vi "471 flame &mq6 (1).vi"() -> ()   [LabVIEW 2017]
panel:
  out "flame indication":bool
  out "Numeric":dbl
  out "dynamic data type":dbl
  out "flame voltage":dbl
  out "mq6 voltage":dbl
  out "Waveform Chart":dynamicdata(graph)
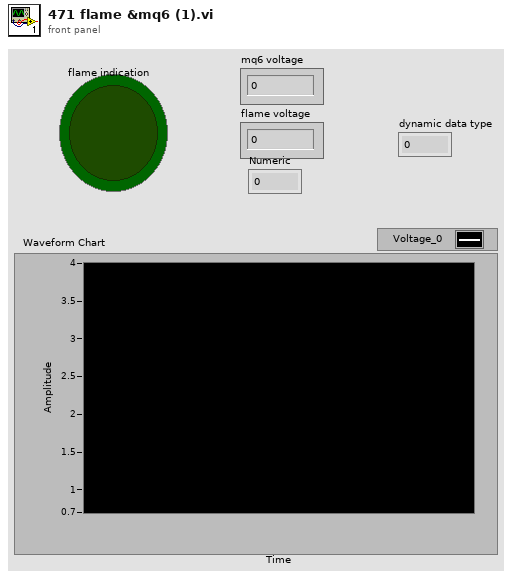
[diagram p1: front panel]
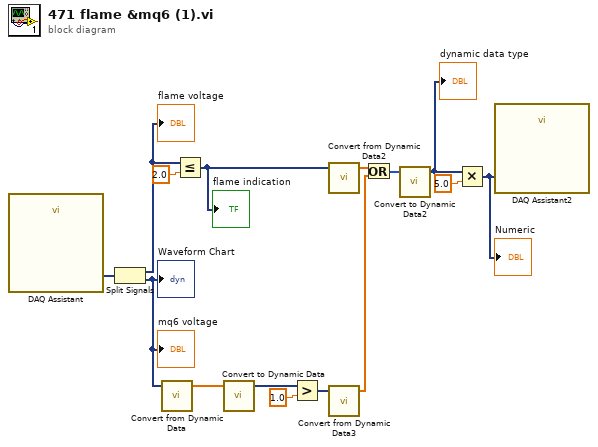
[diagram p0: block diagram]
diagram:
  n1 = call "DAQ Assistant"() -> ("data"=w13:dynamicdata)  [unwired: 16 in, 3 out]
  n2 = Split Signals(w13) -> (w9:dynamicdata, w11:dynamicdata)  [unwired: 2 in]
  "Waveform Chart" <- w11
  "mq6 voltage" <- w11
  "flame voltage" <- w9
  n3 = call "Convert from Dynamic Data"("Dynamic Data Type"=w11) -> ("Array"=w12:dbl[])  [unwired: 3 in]
  n4 = Less Or Equal?(x=w9, y=2.0) -> (x <= y?=w1:dynamicdata)
  "flame indication" <- w1
  n5 = call "Convert to Dynamic Data"("Array"=w12) -> ("Dynamic Data Type"=w14:dynamicdata)  [unwired: 3 in]
  n6 = Greater?(x=w14, y=1.0) -> (0:w8:dynamicdata)
  n7 = call "Convert from Dynamic Data2"("Dynamic Data Type"=w1) -> ("Array"=w7:dbl[])  [unwired: 3 in]
  n8 = call "Convert from Dynamic Data3"("Dynamic Data Type"=w8) -> ("Array"=w6:dbl[])  [unwired: 3 in]
  n9 = Or(x=w7, y=w6) -> (x .or. y?=w5:i32[])
  n10 = call "Convert to Dynamic Data2"("Array"=w5) -> ("Dynamic Data Type"=w4:dynamicdata)  [unwired: 3 in]
  "dynamic data type" <- w4
  n11 = Multiply(x=w4, y=5.0) -> (x*y=w2:dynamicdata)
  "Numeric" <- w2
  n12 = call "DAQ Assistant2"("data"=w2) -> ()  [unwired: 16 in, 3 out]
